vi "module-04-sample-4-1.vi"() -> ()   [LabVIEW 2019]
panel:
  in  "Tab Control":enum32{"Execution", "Logic"}(tab)
  in  "Cycle \nMilliseconds":u32=20 min=10 max=30000 step=10
  in  "AUTO GO Request":bool
  in  "Driver GO Button":bool
  out "Request GO":bool
  in  "IN AUTO MODE":bool
  in  "PERMISSIVE":bool
  in  "Driver STOP Button":bool
  out "Digital State Chart":cluster{dbl, dbl, dbl, dbl, dbl, dbl}(graph)
  # "Training Sample 4.1\nCombinatorial Logic"
  # "F1"
  # "F2"
  # "F3"
  # "F4"
  # "F5"
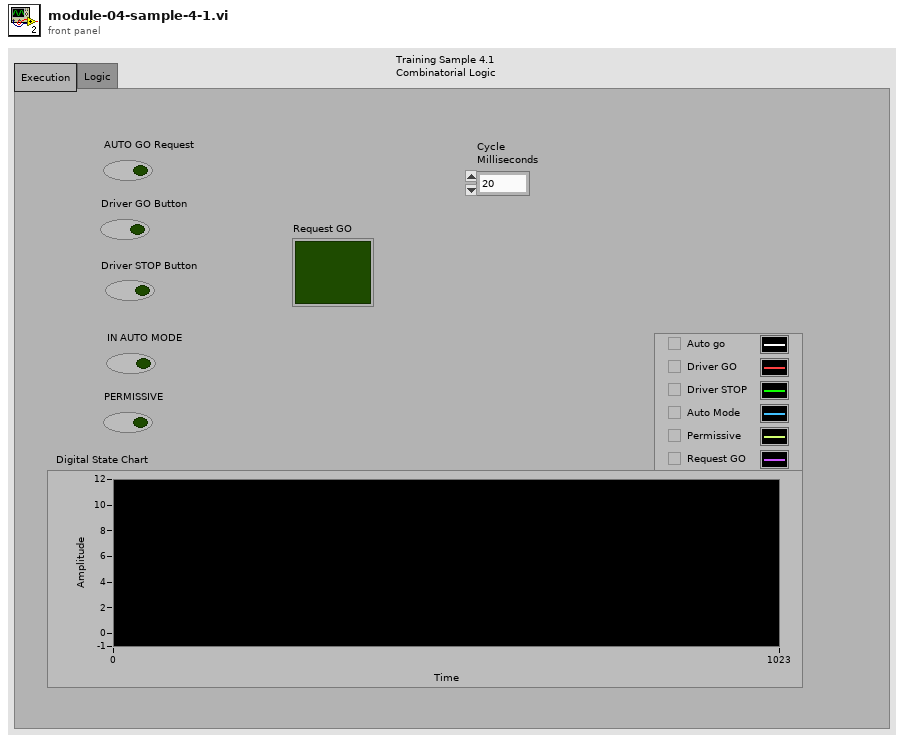
[diagram p1: front panel]
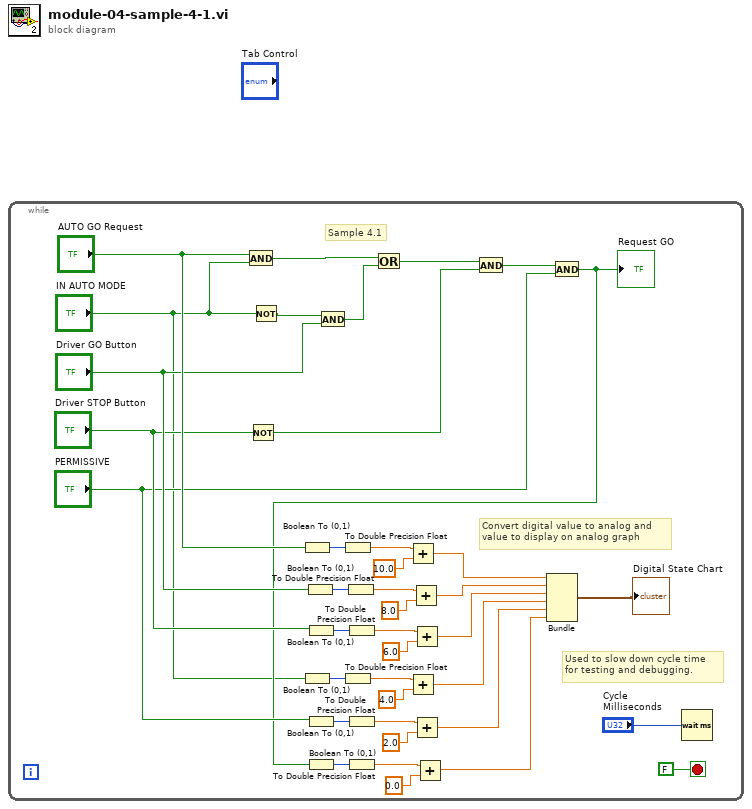
[diagram p0: block diagram]
diagram:
  n1 = while {
    stop <- FALSE stop-if-true
    # "Sample 4.1"
    # "Convert digital value to analog and \nvalue to display on analog graph"
    # "Used to slow down cycle time\nfor testing and debugging."
    n2 = And(x="AUTO GO Request", y="IN AUTO MODE") -> (x .and. y?=w35:bool)
    n3 = Not(x="Driver STOP Button") -> (.not. x?=w36:bool)
    n4 = Not(x="IN AUTO MODE") -> (.not. x?=w38:bool)
    n5 = Boolean To (0,1)(Boolean="AUTO GO Request") -> (0, 1=w31:i16)
    n6 = Boolean To (0,1)(Boolean="IN AUTO MODE") -> (0, 1=w29:i16)
    n7 = Boolean To (0,1)(Boolean="Driver GO Button") -> (0, 1=w26:i16)
    n8 = Boolean To (0,1)(Boolean="Driver STOP Button") -> (0, 1=w23:i16)
    n9 = Boolean To (0,1)(Boolean="PERMISSIVE") -> (0, 1=w20:i16)
    n10 = And(x=w38, y="Driver GO Button") -> (x .and. y?=w34:bool)
    n11 = To Double Precision Float(number=w31) -> (double precision float=w4:dbl)
    n12 = To Double Precision Float(number=w29) -> (double precision float=w28:dbl)
    n13 = To Double Precision Float(number=w26) -> (double precision float=w25:dbl)
    n14 = To Double Precision Float(number=w23) -> (double precision float=w22:dbl)
    n15 = To Double Precision Float(number=w20) -> (double precision float=w19:dbl)
    n16 = Or(x=w35, y=w34) -> (x .or. y?=w33:bool)
    n17 = Add(x=w4, y=10.0) -> (x+y=w3:dbl)
    n18 = Add(x=w28, y=4.0) -> (x+y=w7:dbl)
    n19 = Add(x=w25, y=8.0) -> (x+y=w9:dbl)
    n20 = Add(x=w22, y=6.0) -> (x+y=w8:dbl)
    n21 = Add(x=w19, y=2.0) -> (x+y=w11:dbl)
    n22 = And(x=w33, y=w36) -> (x .and. y?=w37:bool)
    n23 = And(x=w37, y="PERMISSIVE") -> (x .and. y?=w12:bool)
    "Request GO" <- w12
    n24 = Boolean To (0,1)(Boolean=w12) -> (0, 1=w17:i16)
    n25 = To Double Precision Float(number=w17) -> (double precision float=w16:dbl)
    n26 = Add(x=w16, y=0.0) -> (x+y=w10:dbl)
    n27 = Bundle(w3, w9, w8, w7, w11, w10) -> (→"Digital State Chart":cluster{dbl, dbl, dbl, dbl, dbl, dbl})  [unwired: 1 in]
    n28 = Wait (ms)(milliseconds to wait="Cycle \nMilliseconds") -> ()  [unwired: 1 out]
  }
